vi "Destruct.vi"(8 "Error in (no error)":errorcluster, 11 "LogWriterInterface in":refnum<class "LogWriterInterface.lvclass">) -> (0 "Error out":errorcluster, 2 "Array log out":T1[](array[typedef]) {"Priority" items=["EMERGENCY", "ALERT", "CRITICAL", "ERROR", "WARNING", "NOTICE", "INFO", "DEBUG"]})   [LabVIEW 2011, in "LogWriterInterface.lvclass"]
uses:
  LogWriterInterface.lvclass
  Log/LogCluster.ctl
  Log/PrioritiesRing.ctl
  Log/Log.lvclass
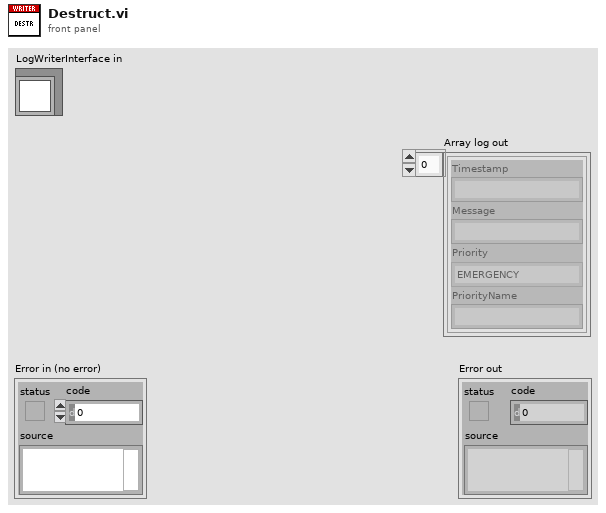
[diagram p1: front panel]
types:
  T1 = typedef "Log.lvclass/LogCluster.ctl" = cluster{"Timestamp":string, "Message":string, "Priority":T2, "PriorityName":string}
  T2 = typedef "Log.lvclass/PrioritiesRing.ctl" = u32
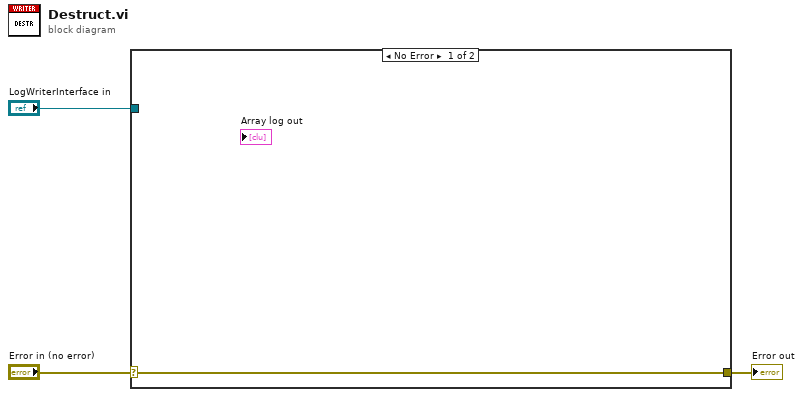
[diagram p0: block diagram]
diagram:
  n1 = case shown="No Error" "Error in (no error)" {
    selector: "Error in (no error)" -> [w4 w5]
    tunnel: [w4 w5] -> w2
    tunnel: "LogWriterInterface in" -> [_ _]
    frame No Error {
    }
    frame Error {
    }
  }
  "Error out" <- w2
